vi "IO Command OUT.vi"() -> ()   [LabVIEW 2011]
panel:
  in  "Status of Output #":dbl[](array[numeric])
  in  "VISA resource name":refnum<visa-resource-name>
  in  "error in (no error)":errorcluster
  out "error out":errorcluster
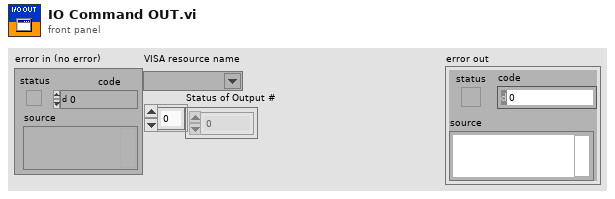
[diagram p1: front panel]
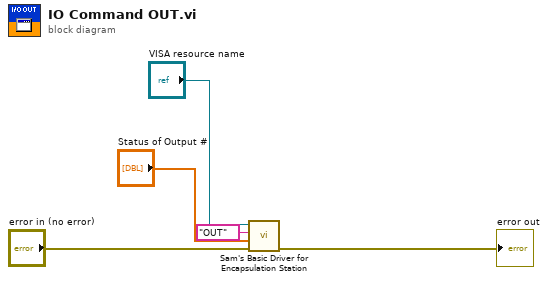
[diagram p0: block diagram]
diagram:
  n1 = call "Sam's Basic Driver for Encapsulation Station.vi"("error in (no error)"="error in (no error)", "Parameter Array"="Status of Output #", "Combo Box"="OUT", "VISA resource name"="VISA resource name") -> ("error out"=→"error out":errorcluster)  [unwired: 5 in, 2 out]
